vi "Setup_Servo.vi"() -> ()   [LabVIEW 2017]
panel:
  in  "Set Servo Position (0 - 180 degrees)":u8(slide)=90 scale=0.0..180.0
  in  "Select Channel":string(combo)="Servo 1"
  in  "stop":bool
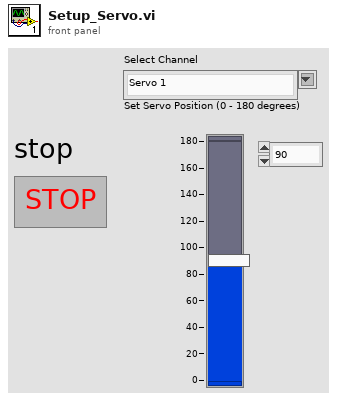
[diagram p1: front panel]
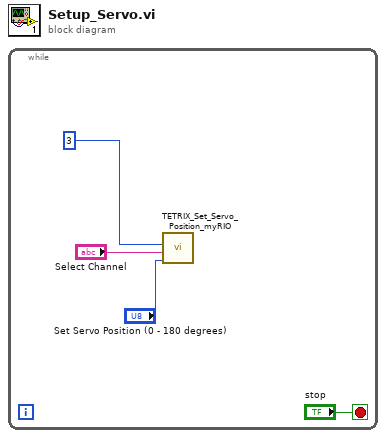
[diagram p0: block diagram]
diagram:
  n1 = while {
    stop <- "stop" stop-if-true
    n2 = call <vilib>:"TETRIX_Set_Servo_Position_myRIO.vi"("Set Servo Position (0 - 180 degrees)"="Set Servo Position (0 - 180 degrees)", "Select Channel"="Select Channel", "Controller ID#  (I2C Address)"=u8 3) -> ()  [unwired: 4 in, 1 out]
  }
